vi "Gear.vi"(9 "Button 0":bool) -> ()   [LabVIEW 2016]
panel:
  out "Switch In Pressed":bool
  out "Switch Out Pressed":bool
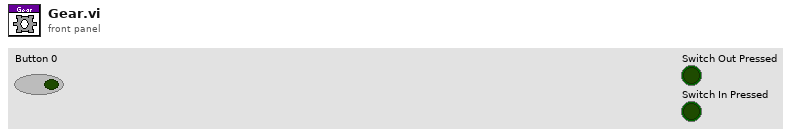
[diagram p1: front panel]
types:
  T1 = typedef "WPI_MotorControlDeviceRef.ctl" = cluster{"DeviceStatus":errorcluster, "Type":T2, "PWM":cluster{"PWM Channel":T3, "DeadBand":T4}, "CAN":cluster{"Device Number":u8, "SetOutput VI Ref":variant, "GetOutput VI Ref":variant, "Enable VI Ref":variant, "Disable VI Ref":variant, "Data":variant}, "Invert":bool}
  T2 = typedef "WPI_MotorControlType.ctl" = enum16{"PWM", "CAN"}
  T3 = typedef "FPGA_DIOPWMChannel.ctl" = enum8{"PWM 0", "PWM 1", "PWM 2", "PWM 3", "PWM 4", "PWM 5", "PWM 6", "PWM 7", "PWM 8", "PWM 9", "PWM MXP 0", "PWM MXP 1", "PWM MXP 2", "PWM MXP 3", "PWM MXP 4", "PWM MXP 5", "PWM MXP 6", "PWM MXP 7", "PWM MXP 8", "PWM MXP 9", "Invalid"}
  T4 = typedef "WPI_PWMDeadband.ctl" = cluster{"Name":string, "maxPositivePwm":i32, "minPositivePwm":i32, "centerPwm":i32, "maxNegativePwm":i32, "minNegativePwm":i32, "angularRange":u16}
  T5 = typedef "WPI_SwitchDevRef.ctl" = cluster{"DevStatus":errorcluster, "DIO Channel":T6, "CntIndex":T7, "Normally Closed":bool}
  T6 = typedef "FPGA_DIOChannel.ctl" = enum8{"DIO 0", "DIO 1", "DIO 2", "DIO 3", "DIO 4", "DIO 5", "DIO 6", "DIO 7", "DIO 8", "DIO 9", "DIO MXP 0", "DIO MXP 1", "DIO MXP 2", "DIO MXP 3", "DIO MXP 4", "DIO MXP 5", "DIO MXP 6", "DIO MXP 7", "DIO MXP 8", "DIO MXP 9", "DIO MXP 10", "DIO MXP 11", "DIO MXP 12", "DIO MXP 13", "DIO MXP 14", "DIO MXP 15", "SPI Port CS1", "SPI Port CS2", "SPI Port CS3", "SPI Port MISO", "SPI Port MOSI", "Invalid"}
  T7 = typedef "FPGA_CounterCtrSystemIndex.ctl" = enum8{"Ctr 0", "Ctr 1", "Ctr 2", "Ctr 3", "Ctr 4", "Ctr 5", "Ctr 6", "Ctr 7", "Invalid"}
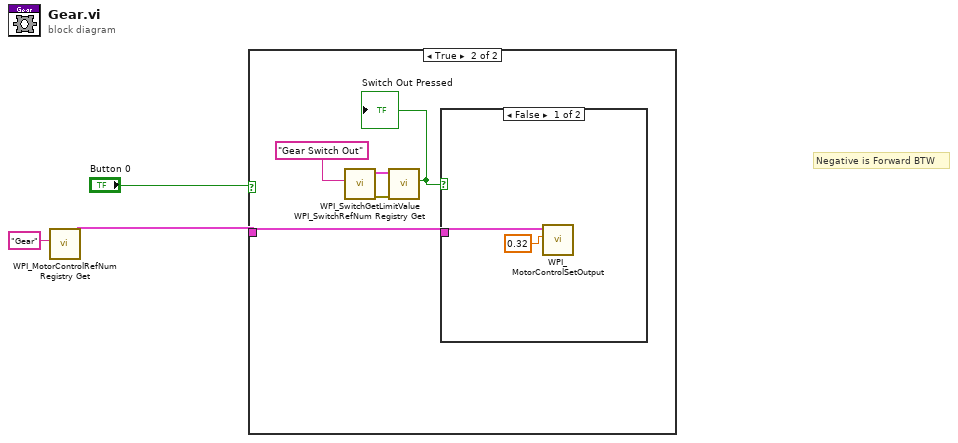
[diagram p0: block diagram]
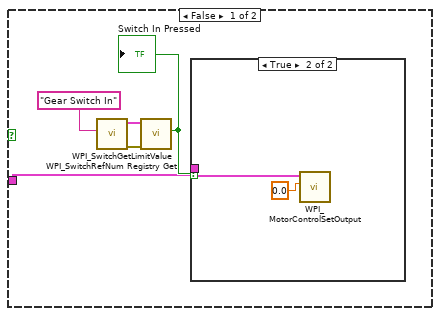
[diagram p2: hidden frame]
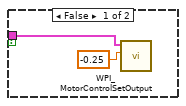
[diagram p3: hidden frame]
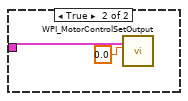
[diagram p4: hidden frame]
diagram:
  # "Negative is Forward BTW"
  n1 = call <vilib>:"WPI_MotorControlRefNum Registry Get.vi"("refnum name"="Gear") -> ("MotorControlDevRef"=w1:T1)  [unwired: 9 in, 1 out]
  n2 = case shown="True" "Button 0" {
    tunnel: w1 -> [w4 w14]
    frame False {
      n3 = call <vilib>:"WPI_SwitchRefNum Registry Get.vi"("refnum name"="Gear Switch In") -> ("error out"=w8:errorcluster, "SwitchDevRef"=w7:T5)  [unwired: 9 in]
      n4 = call <vilib>:"WPI_SwitchGetLimitValue.vi"("error in (no error)"=w8, "SwitchDevRef"=w7) -> ("Switch Pressed"=w5:bool)  [unwired: 7 in, 2 out]
      "Switch In Pressed" <- w5
      n5 = case shown="True" w5 {
        tunnel: w4 -> [w9 w11]
        frame False {
          n6 = call <vilib>:"WPI_MotorControlSetOutput.vi"("Output"=-0.25, "MotorControlDevRef"=w9) -> ()  [unwired: 7 in, 3 out]
        }
        frame True {
          n7 = call <vilib>:"WPI_MotorControlSetOutput.vi"("Output"=0.0, "MotorControlDevRef"=w11) -> ()  [unwired: 7 in, 3 out]
        }
      }
    }
    frame True {
      n8 = call <vilib>:"WPI_SwitchRefNum Registry Get.vi"("refnum name"="Gear Switch Out") -> ("error out"=w17:errorcluster, "SwitchDevRef"=w16:T5)  [unwired: 9 in]
      n9 = call <vilib>:"WPI_SwitchGetLimitValue.vi"("error in (no error)"=w17, "SwitchDevRef"=w16) -> ("Switch Pressed"=w13:bool)  [unwired: 7 in, 2 out]
      "Switch Out Pressed" <- w13
      n10 = case shown="False" w13 {
        tunnel: w14 -> [w19 w21]
        frame False {
          n11 = call <vilib>:"WPI_MotorControlSetOutput.vi"("Output"=0.32, "MotorControlDevRef"=w19) -> ()  [unwired: 7 in, 3 out]
        }
        frame True {
          n12 = call <vilib>:"WPI_MotorControlSetOutput.vi"("Output"=0.0, "MotorControlDevRef"=w21) -> ()  [unwired: 7 in, 3 out]
        }
      }
    }
  }
